vi "AlliGator Create Complementary ROI.vi"(7 "Image Label":string, 8 "Error In":errorcluster, 10 "ROI":T2 {"Contours"."Type" items=["No Selection", "Point", "Line", "Rectangle", "Oval", "Polygon", "Freehand Region", "Annulus", "Unused2", "Unused3", "Broken Line", "Freehand Line", "Rotated Rectangle"]}, 11 "Image":T1) -> (0 "Error Out":errorcluster, 2 "Message":string)   [LabVIEW 2021, in "AlliGator ROIs.lvlib"]
doc: "Computes complementary ROI and adds it to the ROI list."
uses:
  AlliGator ROIs.lvlib
  AlliGator ROI Manager Actions.ctl
  Image/Image.lvlib
  AlliGator Variables List.ctl
  AlliGator Globals, Variables & Constants.lvlib
  Variant/Variant to Data/Variant to Data.lvlib
  <vilib>/ErrorRing/Error Ring.xnode
  <vilib>/Utility/error.llb/Error Cluster From Error Code.vi
  Variant/Variant to Data/Variant to I32.vi
  Image/Named ROI Description.ctl
  AlliGator Source Image ROI Storage [SGL] v3.vi
  AlliGator Phasor Plot Image ROI Storage [SGL] v3.vi
  <vilib>/vision/Image Controls.llb/IMAQ Image.ctl
panel:
  # "see the AlliGator License on the block diagram (Ctrl+E or Window:Show Block Diagram)"
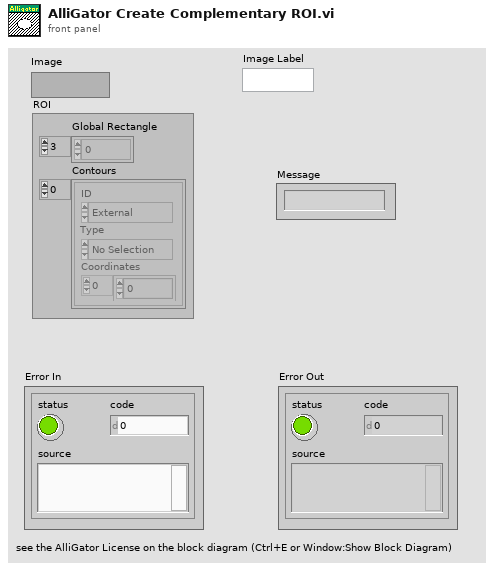
[diagram p1: front panel]
types:
  T1 = typedef "IMAQ Image.ctl" = refnum<image>
  T2 = typedef "ROI Descriptor" = cluster{"Global Rectangle":i32[], "Contours":cluster{"ID":enum32{"External", "Internal"}, "Type":u32, "Coordinates":i32[]}[]}
  T3 = typedef "Image.lvlib/Named ROI Description.ctl" = cluster{"ROI Descriptor":T2, "ROI Name":string, "Overlay Color":u32}
  T4 = typedef "AlliGator Globals, Variables & Constants.lvlib/AlliGator Variables List.ctl" = enum16{"---- GUI ----", "GUI:Initialization Status", "GUI:State Indicators Refnum", "GUI:Original AlliGator Menu Items", "GUI:Current Action Loop State", "GUI:Script in progress", "GUI:Playback", "GUI:Loop Playback", "GUI:Search ROI Used", "GUI:Search ROI", "Decay Graph Max Legend Size", "Intensity Graph Max Legend Size", "Decay Statistics Graph Max Legend Size", "Phasor Graph Max Legend Size", "Phasor Ratio Graph Max Legend Size", "Lifetime Graph Max Legend Size", "---- Files ----", "Files:Export Dataset Frames as Individual Files", "Files:Show Batch Export Help Balloons", "Files:Frames in Dataset", "Files:ptu File Frame Start Indices", "Files:Current Frame in Dataset", "Files:Current Frame Timestamp", "Files:Dataset Loaded", "Files:Dataset Metadata", "Files:Dataset Channel", "Files:Dataset Data Description", "Files:Background Dataset Metadata", "Files:Background Dataset Channel", "Files:Background Dataset Data Description", "Files:Background File Subtraction", "Files:Background File Path", "Files:Background File Pile-up Correction", "Files:Background File Pixel Well Capacity", "Files:Background File Scaling Factor", "Files:Current Dataset Load Settings", "Files:Dataset Path", "Files:ICCD-specific Information", "Files:Macrotime Gate Separation", "------ Python Plugins ------", "Python Plugins:Information", "Python Plugins:Python Session", "Python Plugins:Valid Python Session?", "---- Source Image ----", "Source Image:ROIs", "Source Image:Current ROI", "Source Image:ROI Event Refnum", "X_Source Image Display Range", "X_Source Image Palette Information", "X_Type of Displayed Image", "X_Time Gate Slider", "Source Image:Palette List", "Source Image:Scale", "Source Image:ROI Overlay Color", "Source Image:Overlay to Erase", "Source Image:Is Displayed Image Accumulated", "---- Image Profile Window ----", "Image Profile:Overlay ROI in Source Image", "Image Profile:Window Event Refnum", "Image Profile:IntensityType", "Image Profile:Intensity Average Type", "Image Profile:Intensity-weighted SDV", "Image Profile:Box Profile Type", "Image Profile:Window Open", "Image Profile:Plotted Fit Parameter", "Source Image:White Light Image Modified", "Source Image:Mask Image Modified", "------ Phasor Graph -------", "Phasor Graph:Show Line", "---- Phasor Plot ---", "Phasor Plot:Parameters Changed", "Phasor Plot:FLI Dataset Modified since last Calculation", "Phasor Harmonics Data", "Selected Phasor Harmonics", "Phasor Harmonic Manager Event Refnum", "Phasor Plot:ROIs", "Phasor Plot:Current ROI", "Phasor Plot:ROI Event Refnum", "Phasor Plot:Image Reference Points", "Phasor Plot:Computed", "Phasor Plot:Palette Information", "Phasor Plot:Palette List", "Phasor Ratio Palette Information", "Phasor Ratio Palette List", "Phasor Plot:Image Scale", "Phasor Plot:Image Overlay to Erase", "Phasor Plot:Image Elements to Update", "Current Phasor Plot Calculation Parameters", "Current Phasor Calibration Options", "Phasor Plot:Reset Cumulated Phasor Plot", "Phasor Plot:Reference 1", "Phasor Plot:Lifetime Reference 1", "Phasor Plot:Reference 1 Frequency", "Phasor Plot:Reference 2", "Phasor Plot:Lifetime Reference 2", "Phasor Plot:Reference 2 Frequency", "---- Decay Analysis ----", "Number of Selected Decays to Fit", "LS Fit Results", "LAR Fit Results", "BS Fit Results", "Last Decay Max - Min", "Best Fit Parameters", "Best Fit Parameter Names", "Actual Size X", "Actual Size Y", "Binning X", "Binning Y", "Actual # Gates", "Dataset Number", "Gates to...", "Gates Skipped", "Gates to keep", "Gate Step", "Gate Separation", "Reversed Gates", "Pile-up Correction", "Pixel Well Capacity", "Background Subtracted", "Background Subtraction Method", "Background Definition Range", "Background File (deprecated)", "Number of Dataset Accumulated", "Array of Accumulated Dataset Paths", "Do Averaged Datasets", "Destination File Path", "Process Plot Target", "Use 1/D as Phasor Frequency", "---- Decay Fit Parameter Map -----", "Decay Fit Parameter Map Palette Information", "Decay Fit Parameter Map Palette List", "Local Decay Graph Window Event Refnum", "------- Local Decay Window ---------", "Use normalized IRF for convolution", "----- Miscellaneous ----", "Skippable Dialog Windows Status"}
  T5 = typedef "AlliGator ROIs.lvlib/AlliGator ROI Manager Actions.ctl" = enum16{"Undefined", "Delete Current ROI", "Delete All Unselected ROIs", "Delete Multiple ROIs", "Delete All ROIs", "Swap ROIs", "Insert ROI", "Update Current ROI Descriptor", "Rename Current ROI", "Store New ROI", "Store Multiple ROIs", "Select Next ROI", "Select Previous ROI", "Find Selected ROI", "Show All ROIs", "Update ROI Manager Window", "Merge All ROIs", "Unmerge ROI", "Set Selected ROI by ID"}
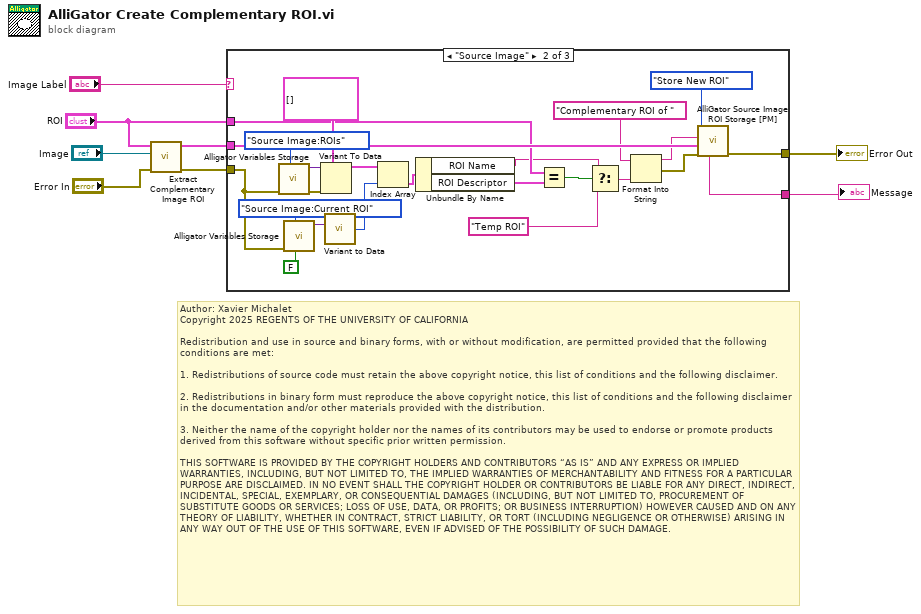
[diagram p0: block diagram]
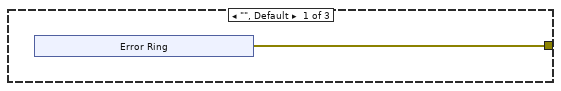
[diagram p2: hidden frame]
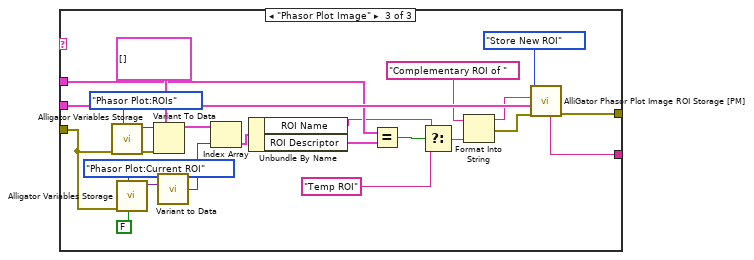
[diagram p3: hidden frame]
diagram:
  # "Author: Xavier Michalet\nCopyright 2025 REGENTS OF THE UNIVERSITY OF CALIFORNIA\n\nRedistribution and use in source and binary forms, with or without modification, are permitted provided that the following conditions are met:\n\n1. Redistributions of source code must retain the above copyright notice, this list of conditions and the following disclaimer.\n\n2. Redistributions in binary form must reproduce the above copyright notice, this list of conditions and the following disclaimer in the documentation and/or other materials provided with the distribution.\n\n3. Neither the name of the copyright holder nor the names of its contributors may be used to endorse or promote products derived from this software without specific prior written permission.\n\nTHIS SOFTWARE IS PROVIDED BY THE COPYRIGHT HOLDERS AND CONTRIBUTORS “AS IS” AND ANY EXPRESS OR IMPLIED WARRANTIES, INCLUDING, BUT NOT LIMITED TO, THE IMPLIED WARRANTIES OF MERCHANTABILITY AND FITNESS FOR A PARTICULAR PURPOSE ARE DISCLAIMED. IN NO EVENT SHALL THE COPYRIGHT HOLDER OR CONTRIBUTORS BE LIABLE FOR ANY DIRECT, INDIRECT, INCIDENTAL, SPECIAL, EXEMPLARY, OR CONSEQUENTIAL DAMAGES (INCLUDING, BUT NOT LIMITED TO, PROCUREMENT OF SUBSTITUTE GOODS OR SERVICES; LOSS OF USE, DATA, OR PROFITS; OR BUSINESS INTERRUPTION) HOWEVER CAUSED AND ON ANY THEORY OF LIABILITY, WHETHER IN CONTRACT, STRICT LIABILITY, OR TORT (INCLUDING NEGLIGENCE OR OTHERWISE) ARISING IN ANY WAY OUT OF THE USE OF THIS SOFTWARE, EVEN IF ADVISED OF THE POSSIBILITY OF SUCH DAMAGE."
  n1 = call "Extract Complementary Image ROI.vi"("error in (no error)"="Error In", "Image Model"="Image", "ROI in"="ROI") -> ("error out"=w5:errorcluster, "Complementary ROI"=w8:T2)  [unwired: 7 in]
  n2 = case shown="\"Source Image\"" "Image Label" {
    tunnel: [w9 w37 w61] -> w3
    tunnel: w8 -> [_ w36 w60]
    tunnel: w5 -> [_ w27 w51]
    tunnel: "ROI" -> [_ w18 w42]
    tunnel: [_ w28 w52] -> w1
    frame "", Default {
      n3 = xnode "Error Ring"() -> ("error out"=w9:errorcluster)
    }
    frame "Source Image" {
      n4 = call "Alligator Variables Storage.vi"("AlliGator Variable"=AlliGator_Variables_List."Source Image:ROIs" ("Alligator Variable"), "Error In"=w27) -> ("Error Out"=w24:errorcluster, "Data out"=w25:variant)  [unwired: 7 in, 1 out]
      n5 = call "Alligator Variables Storage.vi"("Get(F)/Set"=FALSE, "AlliGator Variable"=AlliGator_Variables_List."Source Image:Current ROI" ("Alligator Variable"), "Error In"=w27) -> ("Data out"=w34:variant)  [unwired: 6 in, 2 out]
      n6 = Variant To Data(error in=w24, type=T3[] [] ("ROIs"), Variant=w25) -> (data=w22:T3[])  [unwired: 1 out]
      n7 = call-poly "Variant to Data.vi"("Variant"=w34) -> ("Value"=w21:i32)  [unwired: 8 in]
      n8 = Index Array(array=w22, index=w21) -> (element=w20:T3)
      n9 = Unbundle By Name(w20) -> ("ROI Name"=w16:string, "ROI Descriptor"=w19:T2)
      n10 = Equal?(x=w18, y=w19) -> (x = y?=w17:bool)
      n11 = Select(t=w16, s=w17, f="Temp ROI") -> (s? t:f=w15:string)
      n12 = Format Into String(initial string="Complementary ROI of ", w15) -> (resulting string=w29:string, error out=w30:errorcluster)  [unwired: 2 in]
      n13 = call-poly "AlliGator Source Image ROI Storage [PM].vi"("Error In"=w30, "Current ROI Descriptor"=w36, "Default Name (\"ROI\")"=w29, "Action"=AlliGator_ROI_Manager_Actions."Store New ROI") -> ("Error Out"=w37:errorcluster, "Message"=w28:string)  [unwired: 1 in, 5 out]
    }
    frame "Phasor Plot Image" {
      n14 = call "Alligator Variables Storage.vi"("AlliGator Variable"=AlliGator_Variables_List."Phasor Plot:ROIs" ("Alligator Variable"), "Error In"=w51) -> ("Error Out"=w48:errorcluster, "Data out"=w49:variant)  [unwired: 7 in, 1 out]
      n15 = call "Alligator Variables Storage.vi"("Get(F)/Set"=FALSE, "AlliGator Variable"=AlliGator_Variables_List."Phasor Plot:Current ROI" ("Alligator Variable"), "Error In"=w51) -> ("Data out"=w58:variant)  [unwired: 6 in, 2 out]
      n16 = Variant To Data(error in=w48, type=T3[] [] ("ROIs"), Variant=w49) -> (data=w46:T3[])  [unwired: 1 out]
      n17 = call-poly "Variant to Data.vi"("Variant"=w58) -> ("Value"=w45:i32)  [unwired: 8 in]
      n18 = Index Array(array=w46, index=w45) -> (element=w44:T3)
      n19 = Unbundle By Name(w44) -> ("ROI Name"=w40:string, "ROI Descriptor"=w43:T2)
      n20 = Equal?(x=w42, y=w43) -> (x = y?=w41:bool)
      n21 = Select(t=w40, s=w41, f="Temp ROI") -> (s? t:f=w39:string)
      n22 = Format Into String(initial string="Complementary ROI of ", w39) -> (resulting string=w53:string, error out=w54:errorcluster)  [unwired: 2 in]
      n23 = call-poly "AlliGator Phasor Plot Image ROI Storage [PM].vi"("Error In"=w54, "Current ROI Descriptor"=w60, "Default Name (\"ROI\")"=w53, "Action"=AlliGator_ROI_Manager_Actions."Store New ROI") -> ("Error Out"=w61:errorcluster, "Old ROI Name"=w52:string)  [unwired: 2 in, 4 out]
    }
  }
  "Error Out" <- w3
  "Message" <- w1
